vi "PrintDateTime.vi"(11 "2D Double Array":i32[][](array[numeric])) -> (3 "T button?":bool)   [LabVIEW 2023]
uses:
  <vilib>/Utility/file.llb/Write Delimited Spreadsheet (string).vi
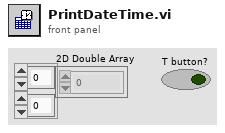
[diagram p1: front panel]
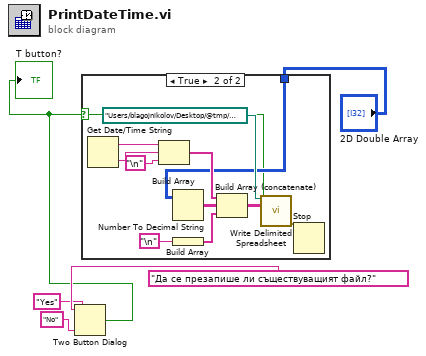
[diagram p0: block diagram]
diagram:
  n1 = Two Button Dialog(message="Да се презапише ли съществуващият файл?", 1:"No" ("F button name (\"Cancel\")"), 2:"Yes" ("T button name (\"OK\")")) -> (T button?=w3:bool)
  "T button?" <- w3
  n2 = case shown="True" w3 {
    selector: w3 -> [_ w8]
    tunnel: "2D Double Array" -> [_ w10]
    frame False {
    }
    frame True {
      n3 = Get Date/Time String() -> (date string=w12:string, time string=w13:string)  [unwired: 3 in]
      n4 = Build Array(w12, w13, "\n") -> (w14:string[])
      n5 = Number To Decimal String(number=w10) -> (decimal integer string=w15:string[][])  [unwired: 1 in]
      n6 = Build Array("\n") -> (w6:string[])
      n7 = Build Array (concatenate)(w14, w15, w6) -> (w16:string[][])
      n8 = call-poly <vilib>:"Write Delimited Spreadsheet.vi"("file path (dialog if empty)"=path "/Users/blagojnikolov/Desktop/@tmp/toto1.txt", "2D data"=w16, "append to file? (new file:F)"=w8) -> ("error out"=w17:errorcluster)  [unwired: 11 in, 1 out]
      n9 = Stop(stop? (T)=w17) -> ()
    }
  }
